vi "filtering.vi"() -> ()   [LabVIEW 2017]
panel:
  out "main signal":waveform(dbl)[](graph) caption="Filtered Signal"
  out "bandpass":dynamicdata(graph) caption="Filtered Signal"
  out "highpass":dynamicdata(graph) caption="Filtered Signal"
  out "lowpass":dynamicdata(graph) caption="Filtered Signal"
  in  "path 3":path
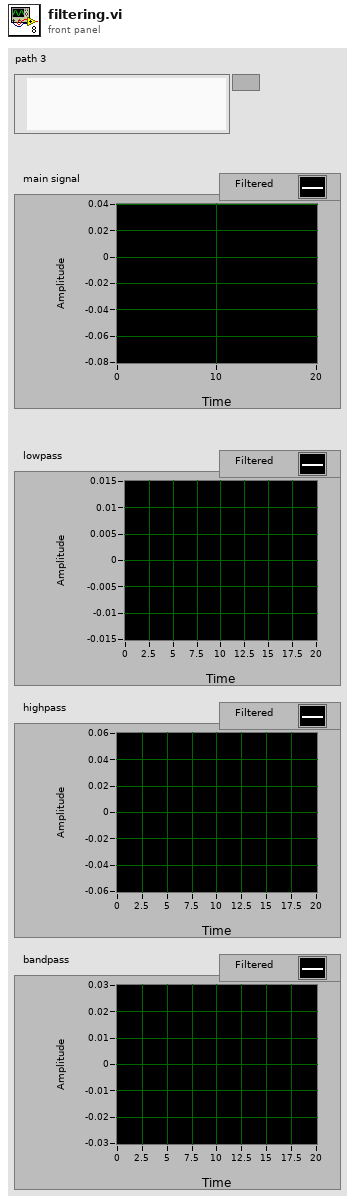
[diagram p1: front panel]
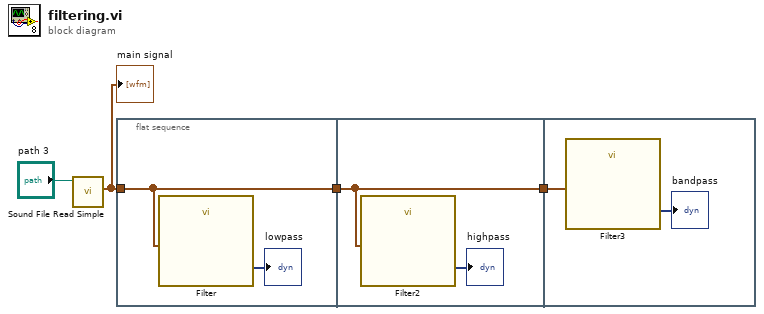
[diagram p0: block diagram]
diagram:
  n1 = call <vilib>:"Sound File Read Simple.vi"("path"="path 3") -> ("data"=w1:waveform(dbl)[])  [unwired: 7 in, 3 out]
  "main signal" <- w1
  n2 = flat-sequence {
    tunnel: w1 -> [w5]
    tunnel: [w5] -> w3
    tunnel: w3 -> [w7]
    tunnel: [w7] -> w2
    tunnel: w2 -> [w10]
    frame #0 {
      n3 = call "Filter"("Signal"=w5) -> ("Filtered Signal"=→"lowpass":dynamicdata)  [unwired: 9 in, 1 out]
    }
    frame #1 {
      n4 = call "Filter2"("Signal"=w7) -> ("Filtered Signal"=→"highpass":dynamicdata)  [unwired: 9 in, 1 out]
    }
    frame #2 {
      n5 = call "Filter3"("Signal"=w10) -> ("Filtered Signal"=→"bandpass":dynamicdata)  [unwired: 9 in, 1 out]
    }
  }
